vi "readVariable_DBL.vi"(6 "ns":u16=2, 8 "error in (no error)":errorcluster, 10 "URL":string, 11 "Client In":refnum<class "Client.lvclass">) -> (0 "error out":errorcluster, 1 "val":dbl, 2 "return type":i32, 3 "Client out":refnum<class "Client.lvclass">)   [LabVIEW 2017, in "opcua.lvlib" / "Client.lvclass"]
uses:
  Client.lvclass
  Client.lvclass/Client.ctl
  opcua.lvlib
  opcua32.dll
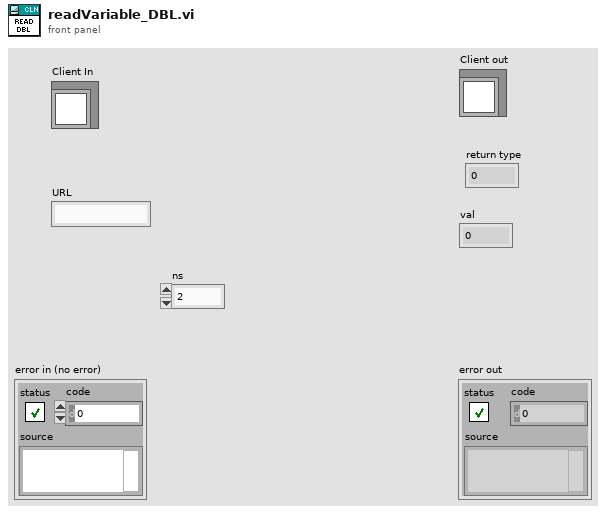
[diagram p1: front panel]
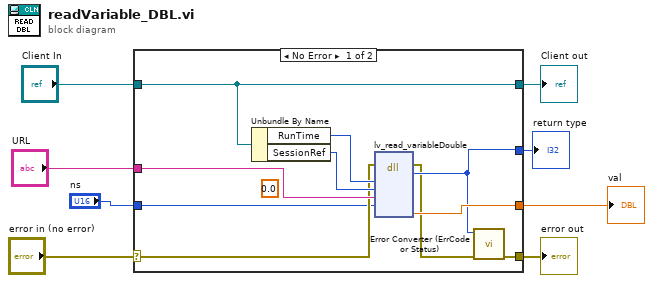
[diagram p0: block diagram]
diagram:
  n1 = case shown="No Error" "error in (no error)" {
    selector: "error in (no error)" -> [w11 w19]
    tunnel: [w18 w19] -> w7
    tunnel: [w15 w20] -> w6
    tunnel: "Client In" -> [w15 w20]
    tunnel: "URL" -> [w14 _]
    tunnel: [w12 _] -> w3
    tunnel: [w13 _] -> w2
    tunnel: "ns" -> [w9 _]
    frame No Error {
      (unwired) 0.0 ("dbl")
      n2 = Unbundle By Name(w15) -> ("RunTime"=w16:u64, "SessionRef"=w17:u64)
      n3 = dll-call lib="C:/Users/108003658/OneDrive - Baker Hughes/Desktop/opcua-0_2_0/opcua-lvlib/opcua*.dll" fn="lv_read_variableDouble"(error in=w11, "runtime"=w16, "client_ref"=w17, "var"=w14, "ns"=w9) -> (error out=w10:errorcluster, "return type"=w12:i32, "val"=w13:dbl)  [unwired: 7 in, 1 out]
      n4 = call "Error Converter (ErrCode or Status).vi"("error in (no error)"=w10, "error code"=w12) -> ("error out"=w18:errorcluster)  [unwired: 9 in]
    }
    frame Error {
    }
  }
  "error out" <- w7
  "Client out" <- w6
  "return type" <- w3
  "val" <- w2
